vi "Streamlined FPGA--130415-2.vi"() -> ()   [LabVIEW 2009]
uses:
  <vilib>/eio/EIONode/EIONode.xnode
  <vilib>/rvi/eio/nirviEIOImplementation/nirviEIOImplementation.xnode
  <vilib>/rvi/eio/common/nirviEmuTemplateMethod_noerrors.vi
  <vilib>/rvi/eio/common/nirviEmuClasses.ctl
  Instance           3 24Saved   Streamlined FPGA .vi
  Instance           4 24Saved   Streamlined FPGA .vi
  Instance           5 24Saved   Streamlined FPGA .vi
  Instance           2 24Saved   Streamlined FPGA .vi
  <vilib>/rvi/DataTransferAndStorage/Container/XNode/niFpgaContainer.xnode
  <vilib>/rvi/interface/RandomDataEmulation/niFpgaRandomDataHandleErrors.vi
  <vilib>/rvi/interface/RandomDataEmulation/nirviRandomDataFPGAFIFO.vi
  <vilib>/rvi/DataTransferAndStorage/Container/Common/niFpgaContainerMethod.ctl
  <vilib>/rvi/DataTransferAndStorage/Container/Common/niFpgaTransferTypeControl.ctl
panel:
  in  "window size":i32
  in  "smooth":bool
  in  "Rec2 Ymin":i32
  in  "Rec2 Xmin":i32
  in  "Rec1 Ymin":i32
  in  "Rec1 Xmin":i32
  in  "Rec2 Ymax":i32
  in  "Rec1 Ymax":i32
  in  "Rec2 Xmax":i32
  in  "Rec1 Xmax":i32
  out "sort!":bool
  in  "Maximum Width":i16
  in  "Maximum Height":i16
  in  "trigger on all":bool
  out "sort pulse":i16
  in  "Baselines":i16[](array[numeric])=[0, 0, 0, 0]
  in  "Sb":i8(ring)=1 items=["PMT1", "PMT2", "PMT3", "PMT4"]
  in  "Sa":i8(ring) items=["PMT1", "PMT2", "PMT3", "PMT4"]
  in  "Sort Case":i8(ring)=1 items=["FP", "Magnitude"]
  out "Full 2":bool
  in  "sort?":bool
  out "Drop counter":u32
  out "sort counter":u32
  in  "PMT to detect drops on":u8
  in  "Minimum Height":i16
  in  "Minimum Width":i16
  in  "Ticks between acquires (Ticks)":u32=200
  in  "Gain 1":i16(slide) scale=-32767.0..32767.0
  in  "Gain 2":i16(slide) scale=-32767.0..32767.0
  in  "Gain 3":i16(slide) scale=-32767.0..32767.0
  in  "Gain 4":i16(slide) scale=-32767.0..32767.0
  in  "amplitude":i16
  in  "1/Frequency \n(ticks)":u32
  in  "Burst \nCycles":i32
  in  "delay [us]":u32=20 min=1 max=8000
  # "Acquisition and Detection"
  # "FP and Sorting Parameters"
  # "Sorting Pulse\nGenerator"
  # "Events"
  # "PMT Controls"
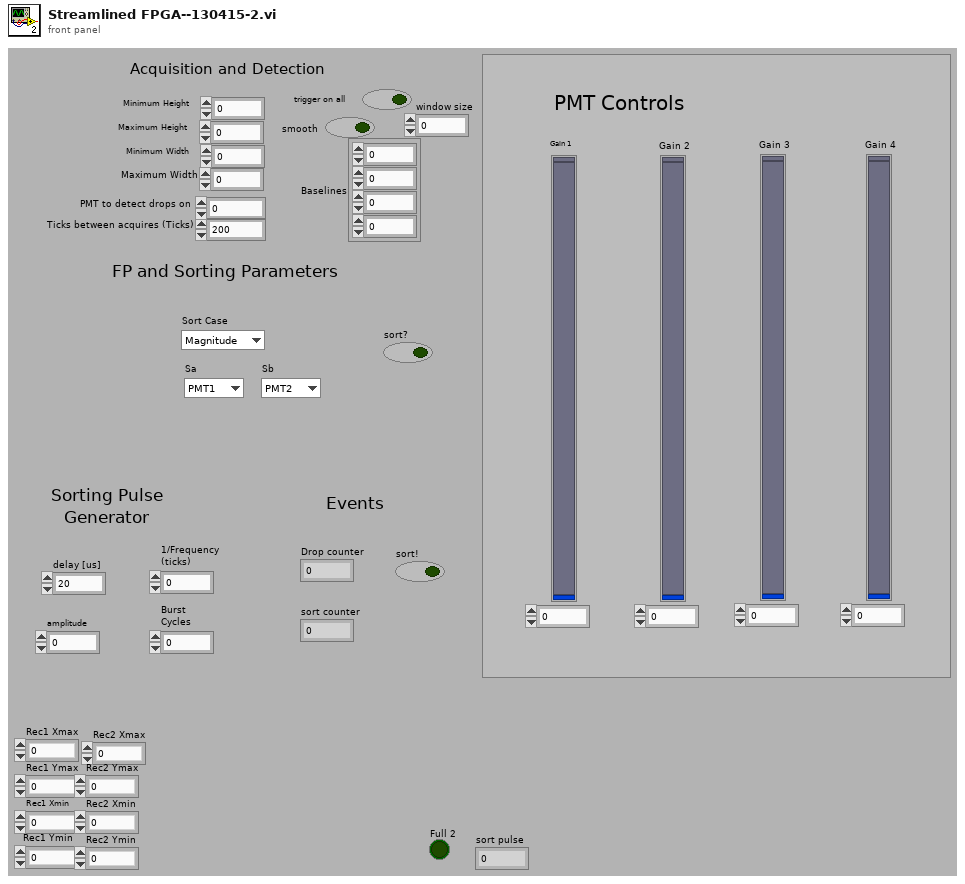
[diagram p1: front panel]
types:
  T1 = typedef "nirviEmuClasses.ctl" = enum16{"IO Read", "IO Write", "Method", "Property Read", "Property Write"}
  T2 = cluster{i32[], i32[], i32[], i32[], i32[], i32[], i32[], i32[]}
  T3 = typedef "niFpgaContainerMethod.ctl" = enum16{"Write", "Read", "Clear", "Get Number of Elements to Write", "Get Number of Elements to Read", "Enable", "Disable", "Flush and Disable", "Get Stream State"}
  T4 = typedef "niFpgaTransferTypeControl.ctl" = enum16{"Target-Scoped", "Host to Target - DMA", "Target to Host - DMA", "Peer to Peer Reader", "Peer to Peer Writer", "Bidirectional"}
  T5 = cluster{"Rec1 Xmax":i32, "Rec1 Ymax":i32, "Rec1 Xmin":i32, "Rec1 Ymin":i32, "Rec2 Xmax":i32, "Rec2 Ymax":i32, "Rec2 Xmin":i32, "Rec2 Ymin":i32}
  T6 = cluster{bool, "max":i16[], "sum":i32[], "time inside":i32, "time outside":i32, "timeoutside-1":i32}
  T7 = cluster{"maxes":i16[], "sums":i32[], "time inside":i32, "time outside":i32}
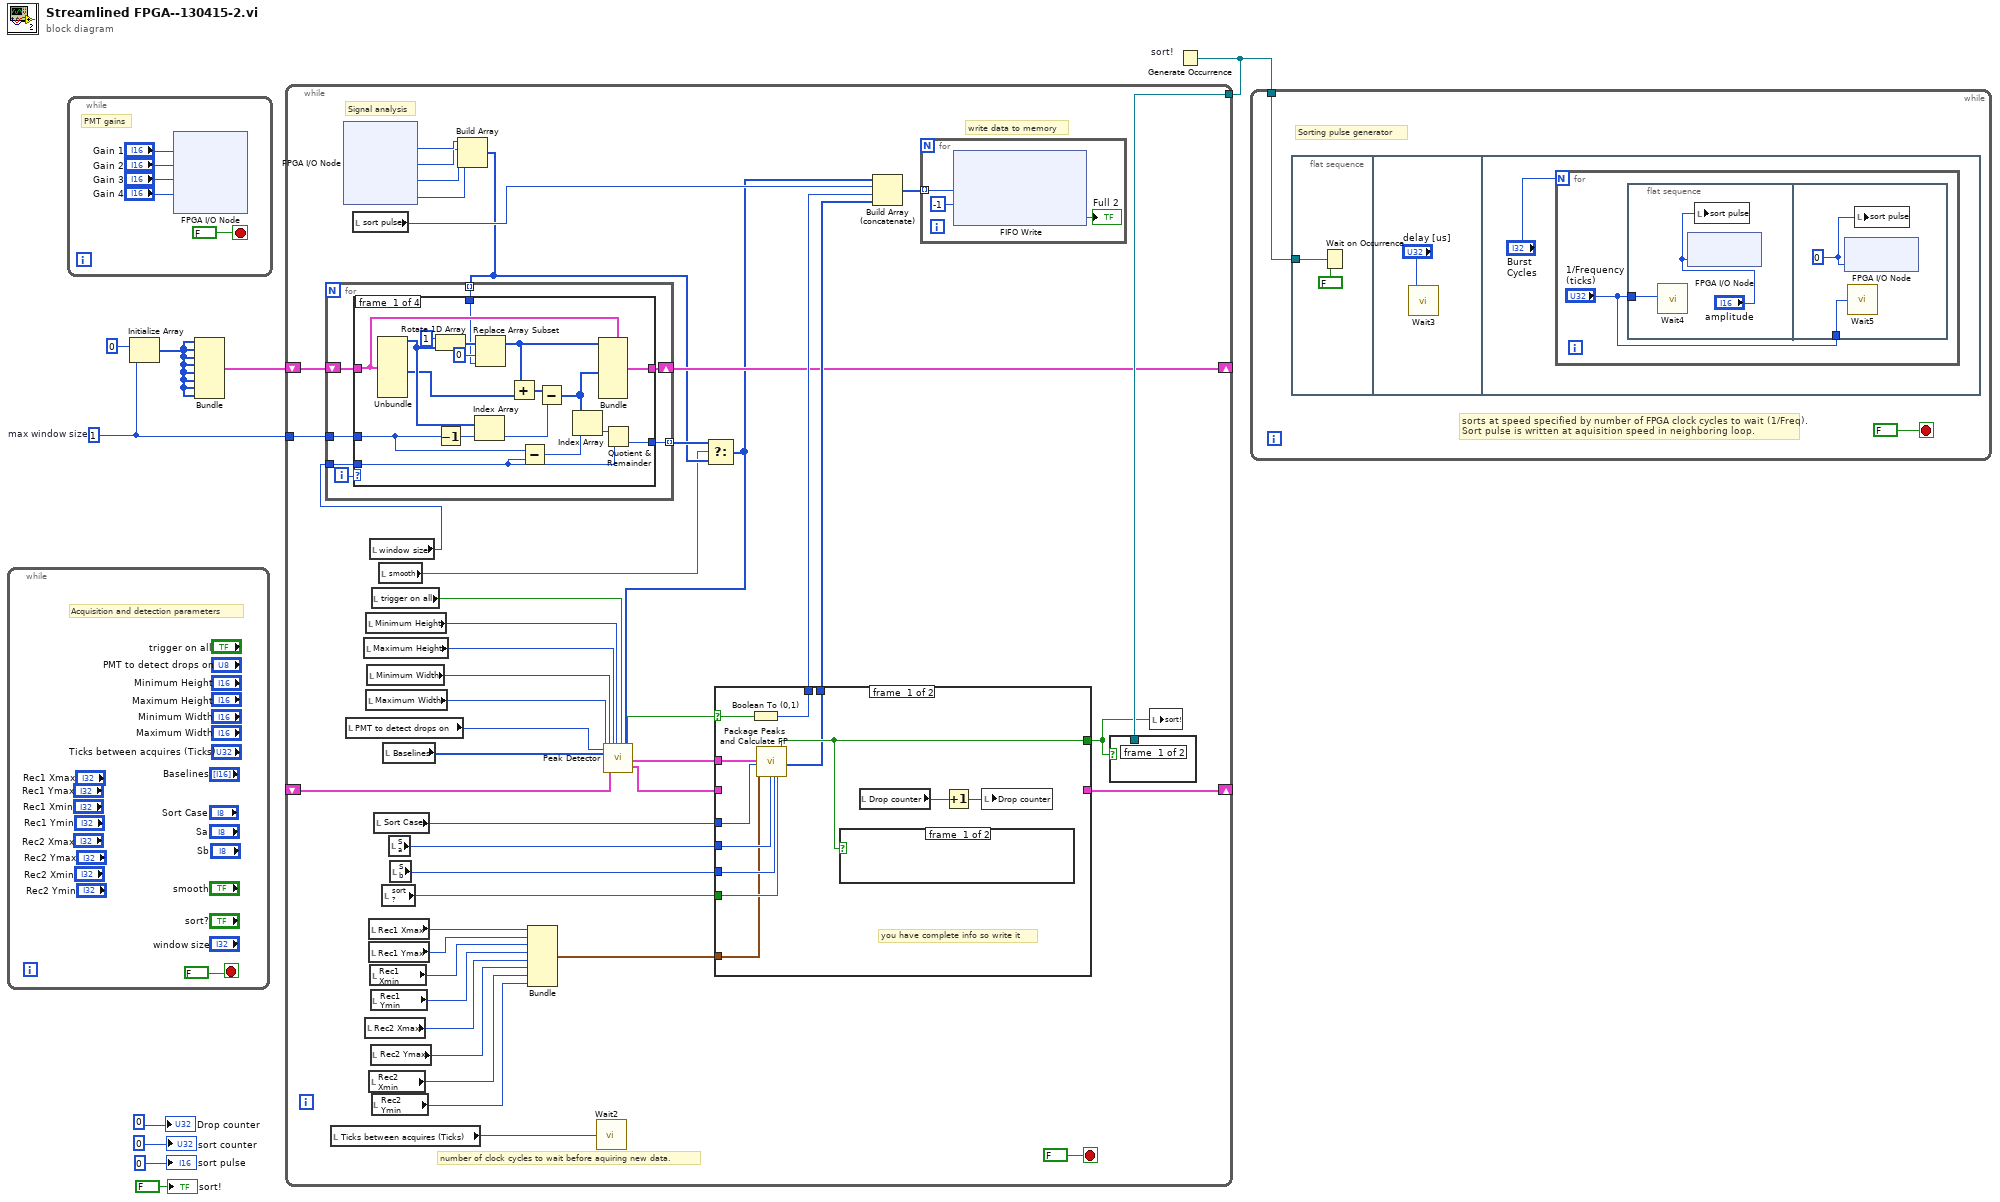
[diagram p0: block diagram]
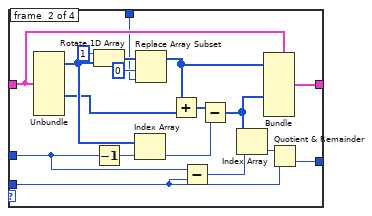
[diagram p2: hidden frame]
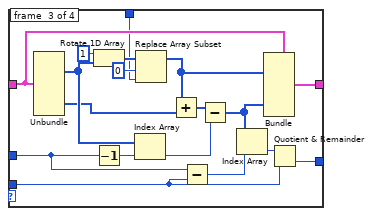
[diagram p3: hidden frame]
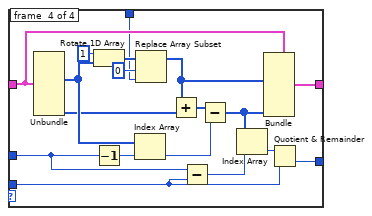
[diagram p4: hidden frame]
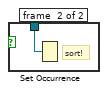
[diagram p5: hidden frame]
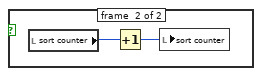
[diagram p6: hidden frame]
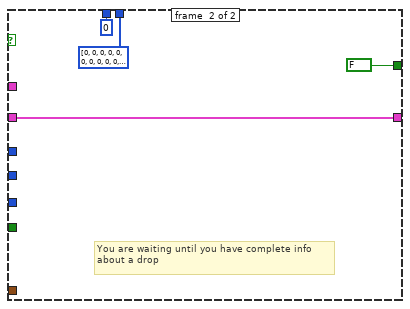
[diagram p7: hidden frame]
diagram:
  w1 = 1  # max window size
  n1 = while {
    stop <- FALSE stop-if-true
    # "Acquisition and detection parameters"
  }
  n2 = while {
    stop <- FALSE stop-if-true
    # "PMT gains"
    n3 = xnode "FPGA I/O Node"("AO0"="Gain 1", "AO1"="Gain 2", "AO2"="Gain 3", "AO3"="Gain 4") -> ()  [unwired: 4 in, 4 out]
  }
  n4 = Initialize Array(0 ("element"), w1) -> (w3:i32[])
  n5 = Bundle(w3, w3, w3, w3, w3, w3, w3, w3) -> (w2:T2)  [unwired: 1 in]
  n6 = Generate Occurrence "sort!"() -> (w9:refnum<k4>)
  n7 = while {
    shift-right: [w103] -> _
    shift-left: _ -> [w90]
    tunnel: w9 -> [w88]
    tunnel: w1 -> [w66]
    shift-right: [w65] -> _
    shift-left: w2 -> [w67]
    stop <- FALSE stop-if-true
    # "number of clock cycles to wait before aquiring new data."
    # "Signal analysis"
    # "write data to memory"
    n8 = local read "Ticks between acquires (Ticks)"() -> (w98:u32)
    n9 = xnode "FPGA I/O Node"() -> ("AI0"=w102:i16, "AI1"=w101:i16, "AI2"=w100:i16, "AI3"=w99:i16)  [unwired: 4 in, 4 out]
    n10 = local read "PMT to detect drops on"() -> (w80:u8)
    n11 = local read "sort pulse"() -> (w87:i16)
    n12 = local read "Maximum Height"() -> (w83:i16)
    n13 = local read "Rec2 Xmax"() -> (w72:i32)
    n14 = local read "Minimum Height"() -> (w84:i16)
    n15 = local read "Maximum Width"() -> (w81:i16)
    n16 = local read "Minimum Width"() -> (w82:i16)
    n17 = local read "Rec1 Xmax"() -> (w76:i32)
    n18 = local read "Rec1 Ymax"() -> (w75:i32)
    n19 = local read "Rec2 Xmin"() -> (w70:i32)
    n20 = local read "window size"() -> (w64:i32)
    n21 = local read "Rec1 Xmin"() -> (w74:i32)
    n22 = local read "Rec1 Ymin"() -> (w73:i32)
    n23 = local read "Rec2 Ymax"() -> (w71:i32)
    n24 = local read "trigger on all"() -> (w89:bool)
    n25 = local read "Rec2 Ymin"() -> (w69:i32)
    n26 = local read "Sort Case"() -> (w97:i8)
    n27 = local read "smooth"() -> (w60:bool)
    n28 = local read "sort?"() -> (w94:bool)
    n29 = local read "Baselines"() -> (w79:i16[])
    n30 = local read "Sa"() -> (w96:i8)
    n31 = local read "Sb"() -> (w95:i8)
    n32 = Build Array(w102, w101, w100, w99) -> (w62:i16[])
    n33 = for {
      tunnel: w66 -> [w110]
      tunnel: [w109] -> w63 mode=indexing
      tunnel: w64 -> [w108]
      tunnel: w62 -> [w106] mode=indexing
      shift-right: [w111] -> w65
      shift-left: w67 -> [w105]
      i -> [w107]
      n34 = case shown="0, Default" w107 {
        tunnel: [w121 w139 w157 w175] -> w111
        tunnel: w105 -> [w122 w140 w158 w176]
        tunnel: w110 -> [w119 w137 w155 w169]
        tunnel: [w116 w134 w152 w166] -> w109
        tunnel: w108 -> [w117 w135 w153 w167]
        tunnel: w106 -> [w120 w138 w156 w170]
        frame #0 {
          n35 = Unbundle(w122) -> (w115:i32[], w113:i32[])  [unwired: 6 out]
          n36 = Rotate 1D Array(1:w115, 2:1 ("n")) -> (0:w128:i32[])
          n37 = Decrement(x=w119) -> (x-1=w126:i32)
          n38 = Index Array(array=w115, index=w126) -> (element=w125:i32)
          n39 = Replace Array Subset(array=w128, new element=w120, index=0 ("n")) -> (w114:i32[])
          n40 = Add(x=w114, y=w113) -> (x+y=w124:i32[])
          n41 = Subtract(x=w119, y=w117) -> (x-y=w123:i32)
          n42 = Subtract(x=w124, y=w125) -> (x-y=w112:i32[])
          n43 = Index Array(array=w112, index=w123) -> (element=w118:i32)
          n44 = Bundle(cluster=w122, w114, w112) -> (w121:T2)  [unwired: 6 in]
          n45 = Quotient & Remainder(x=w118, y=w117) -> (floor(x/y)=w116:i32)  [unwired: 1 out]
        }
        frame #1 {
          n46 = Unbundle(w140) -> (w133:i32[], w131:i32[])  [unwired: 6 out]
          n47 = Rotate 1D Array(1:w133, 2:1 ("n")) -> (0:w146:i32[])
          n48 = Decrement(x=w137) -> (x-1=w144:i32)
          n49 = Index Array(array=w133, index=w144) -> (element=w143:i32)
          n50 = Replace Array Subset(array=w146, new element=w138, index=0 ("n")) -> (w132:i32[])
          n51 = Add(x=w132, y=w131) -> (x+y=w142:i32[])
          n52 = Subtract(x=w137, y=w135) -> (x-y=w141:i32)
          n53 = Subtract(x=w142, y=w143) -> (x-y=w130:i32[])
          n54 = Index Array(array=w130, index=w141) -> (element=w136:i32)
          n55 = Bundle(cluster=w140, w132, w130) -> (w139:T2)  [unwired: 6 in]
          n56 = Quotient & Remainder(x=w136, y=w135) -> (floor(x/y)=w134:i32)  [unwired: 1 out]
        }
        frame #2 {
          n57 = Unbundle(w158) -> (w151:i32[], w149:i32[])  [unwired: 6 out]
          n58 = Rotate 1D Array(1:w151, 2:1 ("n")) -> (0:w164:i32[])
          n59 = Decrement(x=w155) -> (x-1=w162:i32)
          n60 = Index Array(array=w151, index=w162) -> (element=w161:i32)
          n61 = Replace Array Subset(array=w164, new element=w156, index=0 ("n")) -> (w150:i32[])
          n62 = Add(x=w150, y=w149) -> (x+y=w160:i32[])
          n63 = Subtract(x=w155, y=w153) -> (x-y=w159:i32)
          n64 = Subtract(x=w160, y=w161) -> (x-y=w148:i32[])
          n65 = Index Array(array=w148, index=w159) -> (element=w154:i32)
          n66 = Bundle(cluster=w158, w150, w148) -> (w157:T2)  [unwired: 6 in]
          n67 = Quotient & Remainder(x=w154, y=w153) -> (floor(x/y)=w152:i32)  [unwired: 1 out]
        }
        frame #3 {
          n68 = Unbundle(w176) -> (w174:i32[], w173:i32[])  [unwired: 6 out]
          n69 = Rotate 1D Array(1:w174, 2:1 ("n")) -> (0:w182:i32[])
          n70 = Decrement(x=w169) -> (x-1=w180:i32)
          n71 = Index Array(array=w174, index=w180) -> (element=w179:i32)
          n72 = Replace Array Subset(array=w182, new element=w170, index=0 ("n")) -> (w171:i32[])
          n73 = Add(x=w171, y=w173) -> (x+y=w178:i32[])
          n74 = Subtract(x=w169, y=w167) -> (x-y=w177:i32)
          n75 = Subtract(x=w178, y=w179) -> (x-y=w172:i32[])
          n76 = Index Array(array=w172, index=w177) -> (element=w168:i32)
          n77 = Bundle(cluster=w176, w171, w172) -> (w175:T2)  [unwired: 6 in]
          n78 = Quotient & Remainder(x=w168, y=w167) -> (floor(x/y)=w166:i32)  [unwired: 1 out]
        }
      }
    }
    n79 = Bundle("Rec1 Xmax"=w76, "Rec1 Ymax"=w75, "Rec1 Xmin"=w74, "Rec1 Ymin"=w73, "Rec2 Xmax"=w72, "Rec2 Ymax"=w71, "Rec2 Xmin"=w70, "Rec2 Ymin"=w69) -> (w68:T5)  [unwired: 1 in]
    n80 = call "Wait2"("Count(Ticks)"=w98) -> ()  [unwired: 1 out]
    n81 = Select(t=w63, s=w60, f=w62) -> (s? t:f=w61:i32[])
    n82 = call "Peak Detector.vi"("Maximum Width"=w81, "PMT to trigger on (0,1,2,3)"=w80, "Baselines"=w79, "Minimum Width"=w82, "shifts in"=w90, "Maximum Height"=w83, "Minimum Height"=w84, "trigger on all"=w89, "s1,s2,s3,s4"=w61) -> ("peak complete?"=w93:bool, "shifts out"=w91:T6, "peaks data"=w92:T7)  [unwired: 16 in]
    n83 = case shown="True" w93 {
      selector: w93 -> [w294 _]
      tunnel: [_ w305] -> w103
      tunnel: [w292 FALSE ("sort!")] -> w78
      tunnel: w97 -> [w290 _]
      tunnel: w96 -> [w298 _]
      tunnel: w95 -> [w297 _]
      tunnel: w94 -> [w296 _]
      tunnel: w91 -> [_ w305]
      tunnel: w92 -> [w295 _]
      tunnel: [w293 i16 0] -> w85
      tunnel: [w291 i32[] [0, 0, 0, 0, 0, 0, 0, 0, 0, 0, 0, 0] ("M1,M2,M3,M4,S1,S2,S3,S4,Tin,Tout,FP")] -> w77
      tunnel: w68 -> [w289 _]
      frame #0 {
        # "you have complete info so write it"
        n84 = Boolean To (0,1)(Boolean=w294) -> (0, 1=w293:i16)
        n85 = call "Package Peaks and Calculate FP.vi"("peaks data"=w295, "Sort Case"=w290, "Rectangle Positions"=w289, "Sa"=w298, "Sb"=w297, "sort?"=w296) -> ("sort!"=w292:bool, "M1,M2,M3,M4,S1,S2,S3,S4,Tin,Tout,FP,Sort?"=w291:i32[])  [unwired: 14 in, 6 out]
        n86 = case shown="True" w292 {
          frame #0 {
          }
          frame #1 {
            n87 = local read "sort counter"() -> (w302:u32)
            n88 = Increment(x=w302) -> (x+1=w301:u32)
            n89 = local write "sort counter"(w301) -> ()
          }
        }
        n90 = local read "Drop counter"() -> (w300:u32)
        n91 = Increment(x=w300) -> (x+1=w299:u32)
        n92 = local write "Drop counter"(w299) -> ()
      }
      frame #1 {
        # "You are waiting until you have complete info about a drop"
      }
    }
    n93 = Build Array (concatenate)(w61, w87, w85, w77) -> (w86:i32[])
    n94 = for {
      tunnel: w86 -> [w187] mode=indexing
      n95 = xnode ("FIFO Write")("Element"=w187, "Timeout"=-1) -> ("Timed Out?"=→"Full 2":bool)  [unwired: 1 in, 1 out]
    }
    n96 = case shown="True" w78 {
      tunnel: w88 -> [_ w184]
      frame #0 {
      }
      frame #1 {
        # "sort!"
        n97 = Set Occurrence(w184) -> ()
      }
    }
    n98 = local write "sort!"(w78) -> ()
  }
  n99 = while {
    tunnel: w9 -> [w307]
    stop <- FALSE stop-if-true
    # "sorts at speed specified by number of FPGA clock cycles to wait (1/Freq).\nSort pulse is written at aquisition speed in neighboring loop."
    # "Sorting pulse generator"
    n100 = flat-sequence {
      tunnel: w307 -> [w309]
      frame #0 {
        n101 = Wait on Occurrence(1:FALSE ("ignore previous (T)"), 2:w309) -> ()  [unwired: 1 in, 1 out]
      }
      frame #1 {
        n102 = call "Wait3"("Count(uSec)"="delay [us]") -> ()  [unwired: 1 out]
      }
      frame #2 {
        n103 = for {
          N: "Burst \nCycles" -> [_]
          n104 = flat-sequence {
            tunnel: "1/Frequency \n(ticks)" -> [w315]
            tunnel: "1/Frequency \n(ticks)" -> [w328]
            frame #0 {
              n105 = call "Wait4"("Count(Ticks)"=w315) -> ()  [unwired: 1 out]
              n106 = xnode "FPGA I/O Node"("AO4"="amplitude") -> ()  [unwired: 1 in, 1 out]
              n107 = local write "sort pulse"("amplitude") -> ()
            }
            frame #1 {
              w327 = i16 0 ("sort pulse")
              n108 = xnode "FPGA I/O Node"("AO4"=w327) -> ()  [unwired: 1 in, 1 out]
              n109 = call "Wait5"("Count(Ticks)"=w328) -> ()  [unwired: 1 out]
              n110 = local write "sort pulse"(w327) -> ()
            }
          }
        }
      }
    }
  }
  "sort counter" <- u32 0 ("event counter")
  "Drop counter" <- u32 0 ("Drop counter")
  "sort pulse" <- i16 0 ("event counter")
  "sort!" <- FALSE ("sort!")
